vi "Init connection.vi"(8 "error in":errorcluster) -> (0 "error constant":errorcluster, 3 "VISA resource name 2":refnum<visa-resource-name>)   [LabVIEW 2011]
uses:
  <vilib>/Instr/_visa.llb/VISA Configure Serial Port (Instr).vi
panel:
  in  "VISA resource name":refnum<visa-resource-name>="COM8"
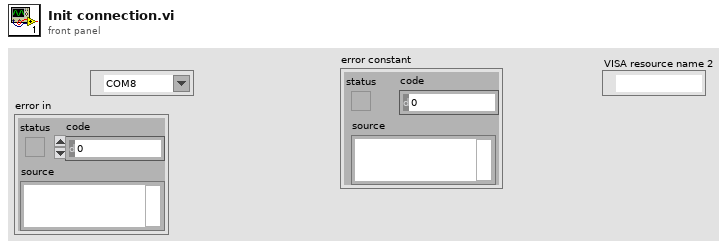
[diagram p1: front panel]
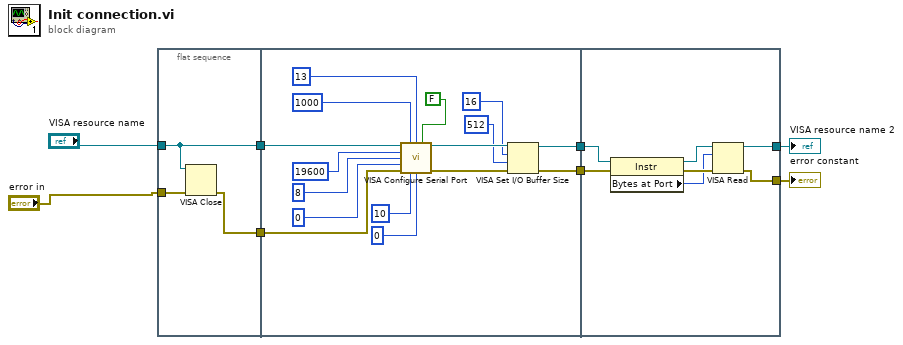
[diagram p0: block diagram]
diagram:
  n1 = flat-sequence {
    tunnel: "VISA resource name" -> [w11]
    tunnel: [w11] -> w7
    tunnel: [w10] -> w2
    tunnel: "error in" -> [w9]
    tunnel: w7 -> [w27]
    tunnel: [w14] -> w6
    tunnel: [w13] -> w5
    tunnel: w2 -> [w12]
    tunnel: w6 -> [w31]
    tunnel: w5 -> [w30]
    tunnel: [w29] -> w4
    tunnel: [w28] -> w3
    frame #0 {
      n2 = VISA Close(VISA resource name=w11, error in (no error)=w9) -> (error out=w10:errorcluster)
    }
    frame #1 {
      n3 = call-poly "VISA Configure Serial Port"("VISA resource name"=w27, "timeout (10sec)"=u32 1000, "termination char\n(0xA = '\\n' = LF)"=u8 13, "Enable Termination\nChar (T)"=FALSE, "baud rate (9600)"=u32 19600, "data bits (8)"=u16 8, "parity (0:none)"=u16 0, "error in (no error)"=w12, "stop bits (10: 1 bit)"=u16 10, "flow control (0:none)"=u16 0) -> ("VISA resource name out"=w17:refnum<visa-resource-name>, "error out"=w18:errorcluster)  [unwired: 4 in]
      n4 = VISA Set I/O Buffer Size(VISA resource name=w17, mask (16)=u16 16, size (4096)=u32 512, error in (no error)=w18) -> (VISA resource name out=w13:refnum<visa-resource-name>, error out=w14:errorcluster)
    }
    frame #2 {
      n5 = property class="Instr"(reference=w30, error in=w31) -> (reference out=w33:refnum<visa-resource-name>, error out=w34:errorcluster, "Bytes at Port"=w32:u32)
      n6 = VISA Read(VISA resource name=w33, byte count=w32, error in (no error)=w34) -> (VISA resource name out=w29:refnum<visa-resource-name>, error out=w28:errorcluster)  [unwired: 2 out]
    }
  }
  "error constant" <- w3
  "VISA resource name 2" <- w4
